vi "Emballage_BDD_sort_SNProduit_2D.vi"(8 "Error in":errorcluster caption="Error in (no error)", 11 "Chaine_Lecteur":string) -> (0 "Error out":errorcluster, 1 "ID_ARTICLE?":bool, 2 "emplacement_CodeBarreFinFixe":string, 3 "SN_PRODUIT":string, 4 "Code 2D?":bool, 5 "ID_ARTICLE":string)   [LabVIEW 2020]
uses:
  Modules/FS/60_FS_Controles/60_FS_SetGet.ctl
panel:
  out "remarque":string
  out "indice":string
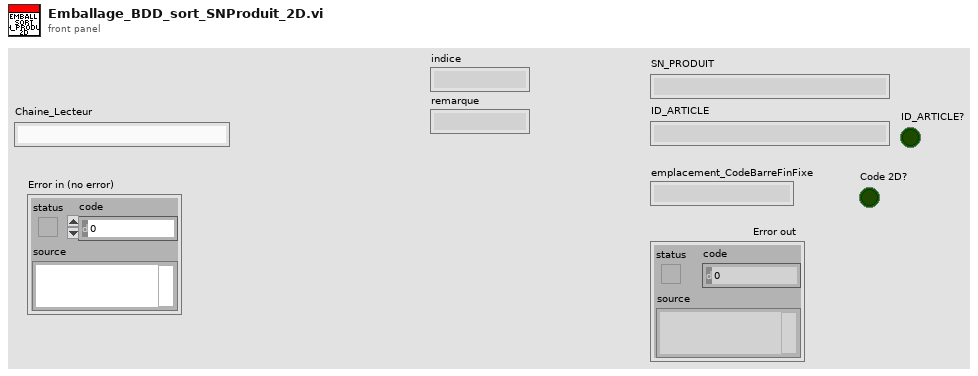
[diagram p1: front panel]
types:
  T1 = typedef "60_FS_SetGet.ctl" = enum16{"set", "get"}
  T2 = typedef "Emballage_BDD_param_Produit.ctl" = cluster{"No_Valve_FAS":string, "suffixe":string, "designation":string, "indice_produit":string, "code_barre_fixe":string, "affiche_code_barre_client":string, "affiche_no_client":string, "Nb_vlve_par_carton":u16, "melange_des_lots_possible":string, "id_article":string, "Indice_Rev":string, "Famille":string, "date":string, "code_barre_fixe_Fin":string, "Longeur_No_Serie":string}
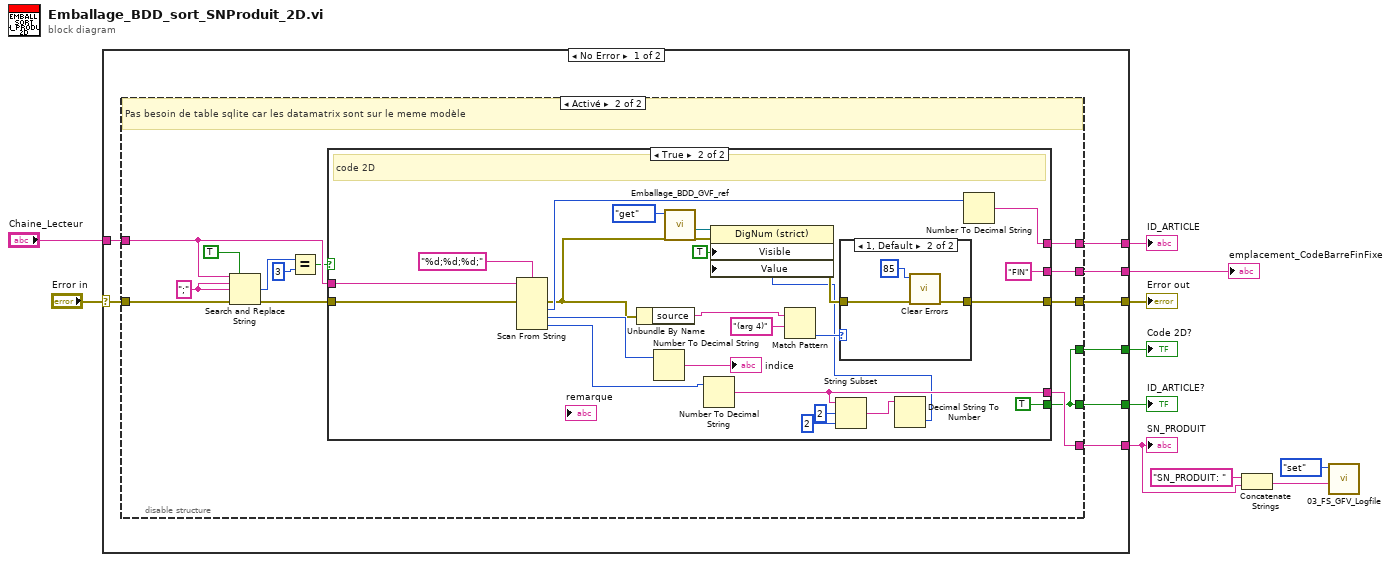
[diagram p0: block diagram]
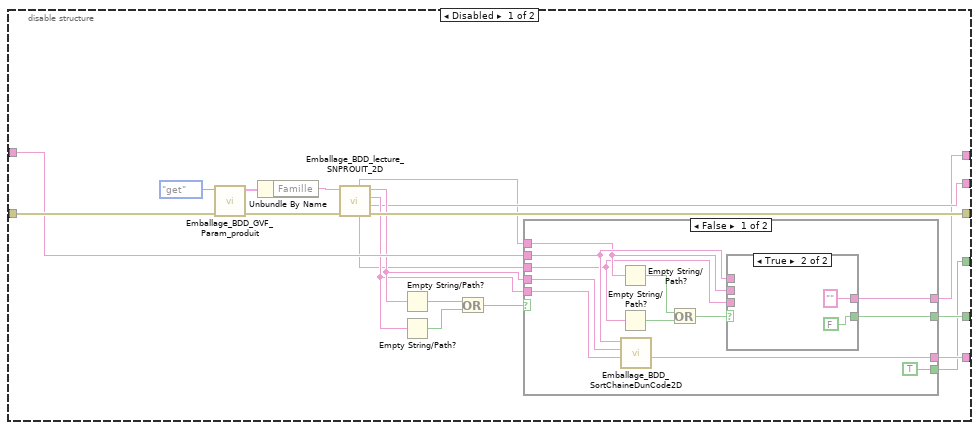
[diagram p2: hidden frame]
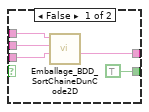
[diagram p3: hidden frame]
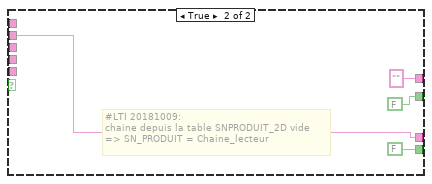
[diagram p4: hidden frame]
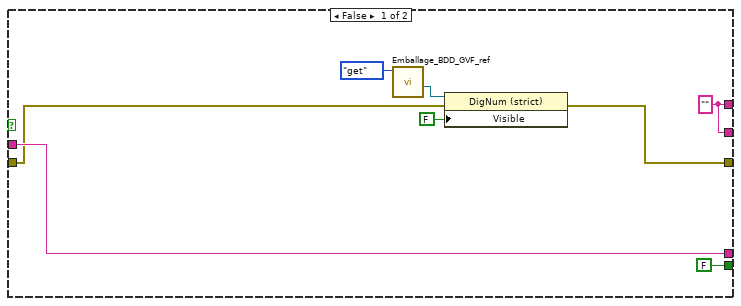
[diagram p5: hidden frame]
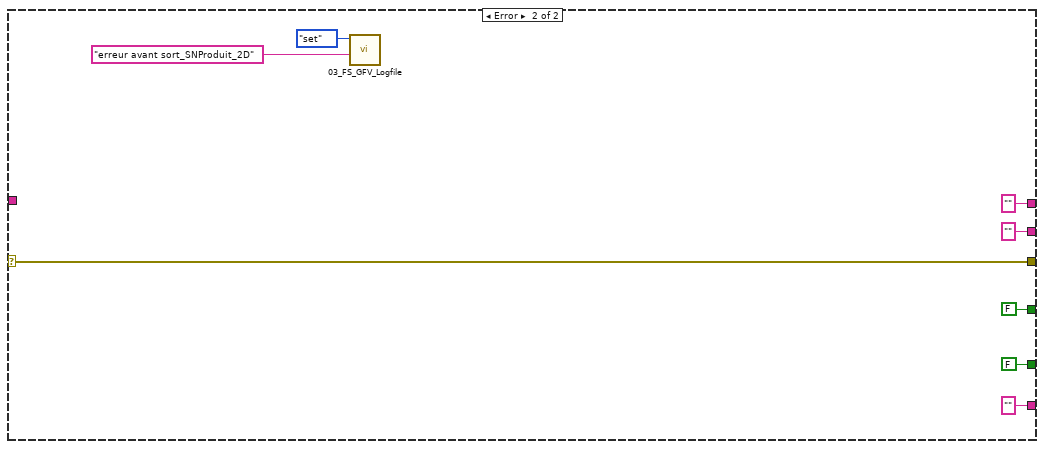
[diagram p7: hidden frame]
diagram:
  n1 = case shown="No Error" "Error in" {
    selector: "Error in" -> [w19 w118]
    tunnel: [w18 w118] -> w10
    tunnel: "Chaine_Lecteur" -> [w17 _]
    tunnel: [w16 "" ("Chaîne IN")] -> w1
    tunnel: [w15 "" ("emplacement_CodeBarreFinFixe")] -> w8
    tunnel: [w14 FALSE] -> w7
    tunnel: [w13 "" ("Chaîne IN")] -> w6
    tunnel: [w12 FALSE] -> w5
    frame No Error {
      n2 = disable-structure shown="Activé" {
        disable-tunnel: w19 -> [w34 w65]
        disable-tunnel: [w33 w64] -> w18
        disable-tunnel: w17 -> [w32 w71]
        disable-tunnel: [w31 w69] -> w16
        disable-tunnel: [w25 w63] -> w15
        disable-tunnel: [w22 w67] -> w14
        disable-tunnel: [w21 w68] -> w13
        disable-tunnel: [w20 w67] -> w12
        frame Disabled {
          n3 = call "Emballage_BDD_GVF_Param_produit.vi"("Error in"=w34, "Énum"=enum16{"set", "get"}."get") -> ("Error out"=w35:errorcluster, "CLS_param_produit"=w37:T2)  [unwired: 6 in, 2 out]
          n4 = Unbundle By Name(w37) -> ("Famille"=w36:string)
          n5 = call "Emballage_BDD_lecture_SNPROUIT_2D.vi"("Error in"=w35, "Famille"=w36) -> ("Error out"=w33:errorcluster, "emplacement_autre"=w25:string, "Fin_SNPRODUIT"=w29:string, "Debut_SNPRODUIT"=w30:string, "FIN_IDARTICLE"=w23:string, "Debut_IDARTICLE"=w24:string)  [unwired: 4 in]
          n6 = Empty String/Path?(string/path=w30) -> (empty?=w27:bool)
          n7 = Empty String/Path?(string/path=w29) -> (empty?=w28:bool)
          n8 = Or(x=w27, y=w28) -> (x .or. y?=w26:bool)
          n9 = case shown="False" w26 {
            tunnel: w30 -> [w50 _]
            tunnel: w29 -> [w49 _]
            tunnel: w32 -> [w42 w61]
            tunnel: [w48 w61] -> w31
            tunnel: w24 -> [w41 _]
            tunnel: w23 -> [w40 _]
            tunnel: [w44 FALSE] -> w22
            tunnel: [w43 ""] -> w21
            tunnel: [TRUE FALSE] -> w20
            frame False {
              n10 = Empty String/Path?(string/path=w41) -> (empty?=w46:bool)
              n11 = Empty String/Path?(string/path=w40) -> (empty?=w45:bool)
              n12 = call "Emballage_BDD_SortChaineDunCode2D.vi"("Fin_CHAINE"=w49, "Debut_CHAINE"=w50, "Chaine_Lecteur"=w42) -> ("Chaîne OUT"=w48:string)  [unwired: 8 in]
              n13 = Or(x=w46, y=w45) -> (x .or. y?=w47:bool)
              n14 = case shown="True" w47 {
                tunnel: [TRUE FALSE] -> w44
                tunnel: [w54 "" ("Chaîne OUT")] -> w43
                tunnel: w42 -> [w53 _]
                tunnel: w41 -> [w52 _]
                tunnel: w40 -> [w51 _]
                frame False {
                  n15 = call "Emballage_BDD_SortChaineDunCode2D.vi"("Fin_CHAINE"=w51, "Debut_CHAINE"=w52, "Chaine_Lecteur"=w53) -> ("Chaîne OUT"=w54:string)  [unwired: 8 in]
                }
                frame True {
                }
              }
            }
            frame True {
              # "#LTI 20181009:\nchaine depuis la table SNPRODUIT_2D vide\n=> SN_PRODUIT = Chaine_lecteur"
            }
          }
        }
        frame Enabled {
          w74 = ";" ("chaîne recherchée")
          # "Pas besoin de table sqlite car les datamatrix sont sur le meme modèle"
          n16 = Search and Replace String(replace all?=TRUE ("tout remplacer ? (F)"), input string=w71, search string=w74, replace string=w74, error in=w65) -> (number of replacements=w73:i32, error out=w66:errorcluster)  [unwired: 3 in, 2 out]
          n17 = Equal?(x=w73, y=3) -> (x = y?=w70:bool)
          n18 = case shown="True" w70 {
            tunnel: w71 -> [w82 w105]
            tunnel: [w82 w88] -> w69
            tunnel: [w80 w98] -> w68
            tunnel: [FALSE TRUE] -> w67
            tunnel: w66 -> [w75 w100]
            tunnel: [w76 w94] -> w64
            tunnel: [w80 "FIN" ("emplacement_autre")] -> w63
            frame False {
              w80 = ""
              n19 = call "Emballage_BDD_GVF_ref.vi"("Énum"=enum16{"set", "get"}."get") -> ("Refnum NumSem OUT"=w78:refnum<vi>)  [unwired: 9 in, 1 out]
              n20 = property class="DigNum (strict)"(reference=w78, error in=w75, "Visible"=FALSE) -> (error out=w76:errorcluster)  [unwired: 1 out]
            }
            frame True {
              # "code 2D"
              n21 = Scan From String(format string="%d;%d;%d;" ("chaîne de format"), input string=w105, error in=w100) -> (error out=w89:errorcluster, output 1=w104:i32, output 2=w103:i32, output 3=w102:i32)  [unwired: 4 in, 2 out]
              n22 = Unbundle By Name(w89) -> ("source"=w96:string)
              n23 = Number To Decimal String(number=w103) -> (decimal integer string=→"indice":string)  [unwired: 1 in]
              n24 = call "Emballage_BDD_GVF_ref.vi"("Énum"=enum16{"set", "get"}."get") -> ("Refnum NumSem OUT"=w91:refnum<vi>)  [unwired: 9 in, 1 out]
              n25 = Number To Decimal String(number=w102) -> (decimal integer string=w88:string)  [unwired: 1 in]
              n26 = Match Pattern(string=w96, regular expression="(arg 4)" ("expression régulière")) -> (offset past match=w93:i32)  [unwired: 1 in, 3 out]
              n27 = String Subset(string=w88, offset (0)=2, length (rest)=2 ("longueur (reste)")) -> (substring=w85:string)
              n28 = Decimal String To Number(string=w85) -> (number=w83:i32)  [unwired: 2 in, 1 out]
              n29 = property class="DigNum (strict)"(reference=w91, error in=w89, "Visible"=TRUE, "Value"=w83) -> (error out=w84:errorcluster)  [unwired: 1 out]
              n30 = case shown="1, Default" w93 {
                tunnel: w84 -> [w107 w110]
                tunnel: [w107 w109] -> w94
                frame -1 {
                }
                frame 1, Default {
                  n31 = call <vilib>:"Clear Errors.vi"("error in (no error)"=w110, "specific error code to clear (0: all)"=85) -> ("error out"=w109:errorcluster)  [unwired: 4 in, 1 out]
                }
              }
              n32 = Number To Decimal String(number=w104) -> (decimal integer string=w98:string)  [unwired: 1 in]
            }
          }
        }
      }
    }
    frame Error {
      n33 = call "03_FS_GFV_Logfile.vi"("Chaîne"="erreur avant sort_SNProduit_2D", "States"=60_FS_SetGet."set") -> ()  [unwired: 8 in, 2 out]
    }
  }
  "Error out" <- w10
  "SN_PRODUIT" <- w1
  "emplacement_CodeBarreFinFixe" <- w8
  "ID_ARTICLE?" <- w7
  "ID_ARTICLE" <- w6
  "Code 2D?" <- w5
  n34 = Concatenate Strings("SN_PRODUIT: " ("chaîne"), w1) -> (w3:string)
  n35 = call "03_FS_GFV_Logfile.vi"("Chaîne"=w3, "States"=60_FS_SetGet."set") -> ()  [unwired: 8 in, 2 out]
